vi "Status Alarm Condition.vi"(0 "VISA resource name":refnum<visa-resource-name>, 7 "Input (1)":dbl=1.0 min=1.0 max=8.0 step=1.0, 11 "error in (no error)":errorcluster) -> (4 "VISA resource name out":refnum<visa-resource-name>, 6 "Alarm High Status":bool, 8 "Alarm Low Status":bool, 10 "Beeper Status":bool, 15 "error out":errorcluster)   [LabVIEW 2012, in "Lake Shore Cryotronics 218.lvlib"]
doc: "This VI indicates the status of the 218 alarm functions. Indicators are provided for both high and low alarm status for a selected input. System beeper status is also indicated."
uses:
  <instrlib>/Lake Shore Cryotronics 218/Lake Shore Cryotronics 218.lvlib
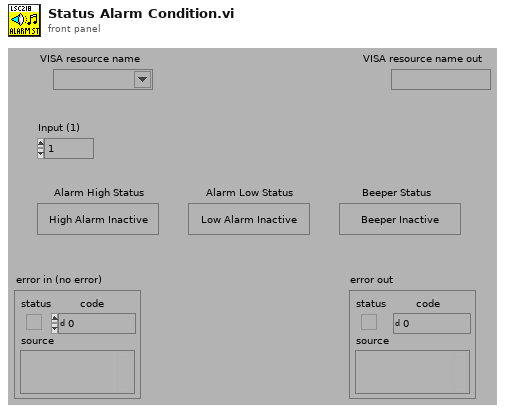
[diagram p1: front panel]
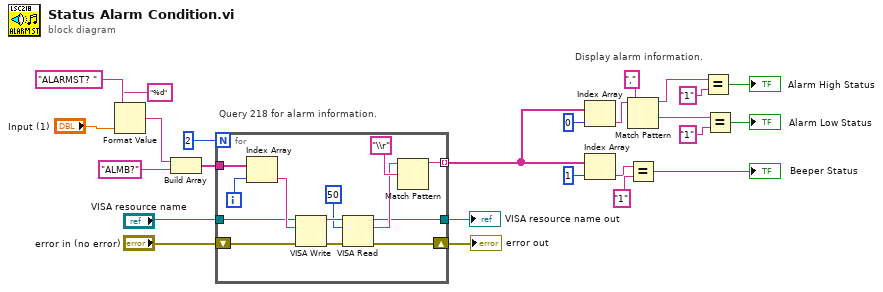
[diagram p0: block diagram]
diagram:
  # "Query 218 for alarm information."
  # "Display alarm information."
  n1 = Format Value(string ("")="ALARMST? ", format string="%d", value (0)="Input (1)") -> (output string=w13:string)
  n2 = Build Array(w13, "ALMB?") -> (w20:string[])
  n3 = for {
    N: 2 -> [_]
    tunnel: [w34] -> w12 mode=indexing
    shift-right: [w31] -> w2
    shift-left: "error in (no error)" -> [w32]
    tunnel: [w27] -> w1
    tunnel: w20 -> [w29]
    tunnel: "VISA resource name" -> [w26]
    i -> [w33]
    n4 = Index Array(array=w29, index=w33) -> (element=w30:string)
    n5 = VISA Write(VISA resource name=w26, write buffer=w30, error in (no error)=w32) -> (VISA resource name out=w38:refnum<visa-resource-name>, error out=w37:errorcluster)  [unwired: 1 out]
    n6 = VISA Read(VISA resource name=w38, byte count=50, error in (no error)=w37) -> (VISA resource name out=w27:refnum<visa-resource-name>, read buffer=w35:string, error out=w31:errorcluster)  [unwired: 1 out]
    n7 = Match Pattern(string=w35, regular expression="\\r") -> (before substring=w34:string)  [unwired: 1 in, 3 out]
  }
  "VISA resource name out" <- w1
  "error out" <- w2
  n8 = Index Array(array=w12, index=0) -> (element=w10:string)
  n9 = Index Array(array=w12, index=1) -> (element=w17:string)
  n10 = Match Pattern(string=w10, regular expression=",") -> (before substring=w6:string, after substring=w5:string)  [unwired: 1 in, 2 out]
  n11 = Equal?(x=w17, y="1") -> (x = y?=→"Beeper Status":bool)
  n12 = Equal?(x=w6, y="1") -> (x = y?=→"Alarm High Status":bool)
  n13 = Equal?(x=w5, y="1") -> (x = y?=→"Alarm Low Status":bool)
